vi "Target Deterministic Tasks.vi"(6 "rt fifo":refnum<k33>, 8 "Start Time (uSec)":u32) -> (0 "Stop":bool)   [LabVIEW 2018]
uses:
  Target Logging Cluster.ctl
  Target Sensors.ctl
  Target Telemetry Cluster.ctl
  COBRA-Libraries/Data Logging/COBRA Logging and Loop Timing Library.lvlib
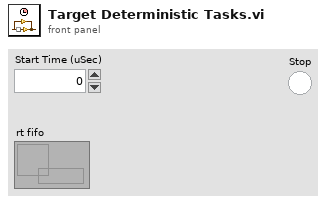
[diagram p1: front panel]
types:
  T1 = typedef "Target Logging Cluster.ctl" = cluster{"Valid for Logging?":bool, "Target Sensors":T2}
  T2 = typedef "Target Sensors.ctl" = cluster{"Raw Cable Force (N)":dbl, "Prosthesis Angle (deg)":dbl, "Main Clock Line (s)":dbl}
  T3 = enum16{"Manual Button Press", "External Voltage"}
  T4 = typedef "Target Telemetry Cluster.ctl" = cluster{"Target Sensors":T2}
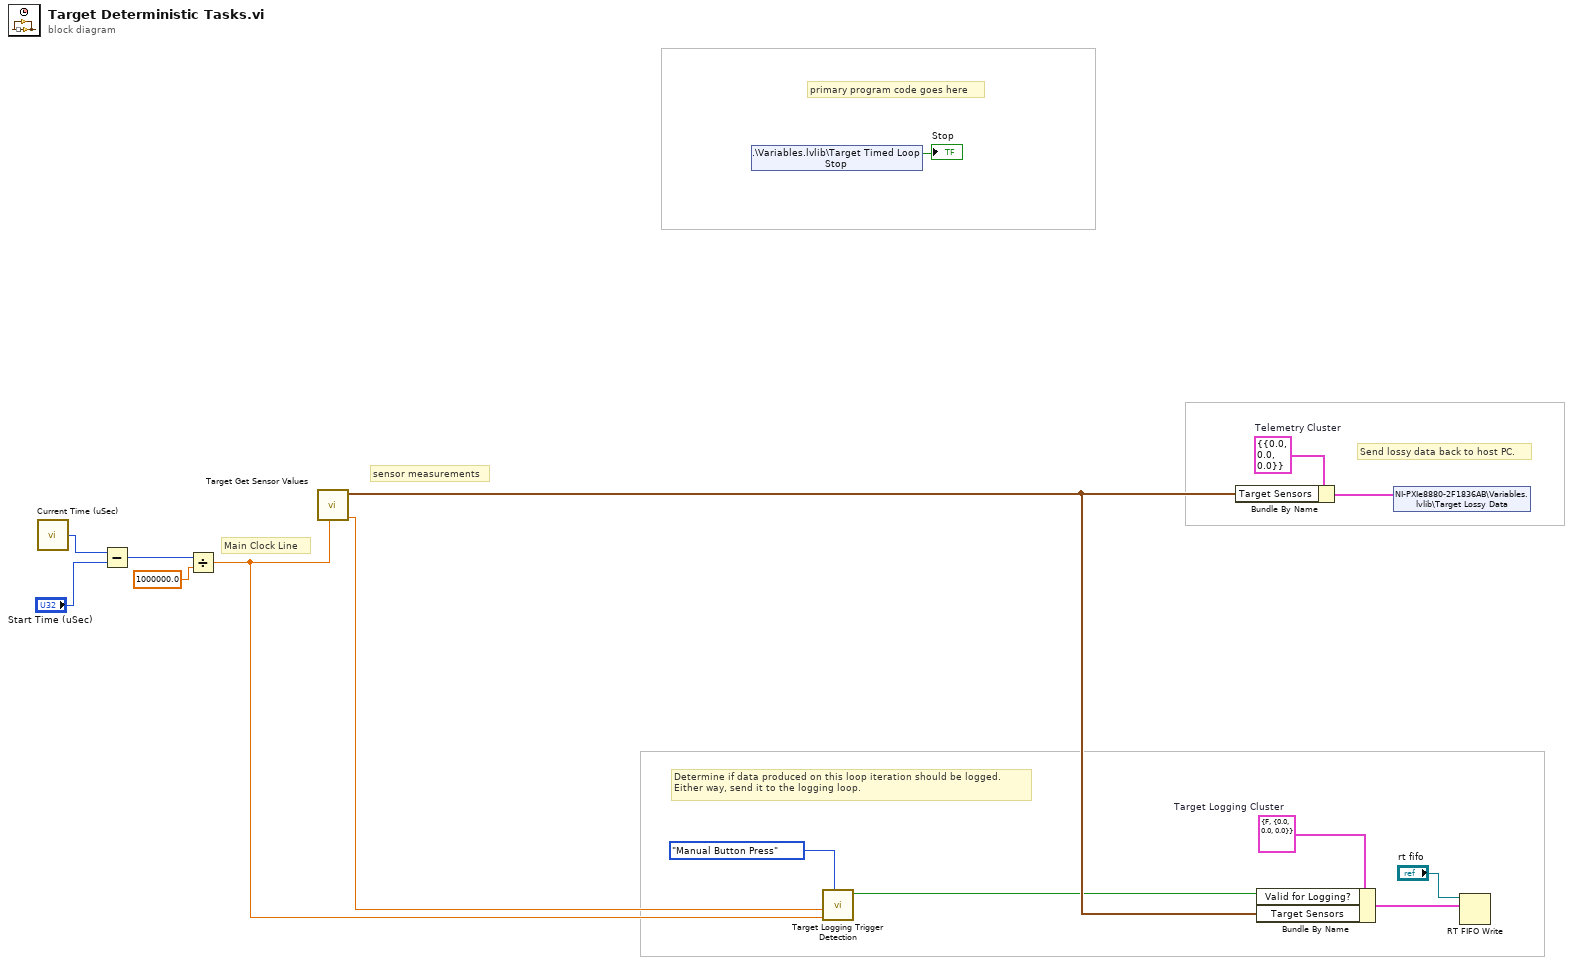
[diagram p0: block diagram]
diagram:
  w6 = T1 {"Valid for Logging?"=FALSE, "Target Sensors"={"Raw Cable Force (N)"=0.0, "Prosthesis Angle (deg)"=0.0, "Main Clock Line (s)"=0.0}}  # Target Logging Cluster
  w13 = T4 {"Target Sensors"={"Raw Cable Force (N)"=0.0, "Prosthesis Angle (deg)"=0.0, "Main Clock Line (s)"=0.0}}  # Telemetry Cluster
  # "primary program code goes here"
  # "sensor measurements"
  # "Main Clock Line"
  # "Send lossy data back to host PC."
  # "Determine if data produced on this loop iteration should be logged.\nEither way, send it to the logging loop."
  n1 = call "Current Time (uSec)"() -> ("Tick Count(uSec)"=w9:u32)
  n2 = Subtract(x=w9, y="Start Time (uSec)") -> (x-y=w11:u32)
  n3 = Divide(x=w11, y=1000000.0) -> (x/y=w4:dbl)
  n4 = call "Target Get Sensor Values.vi"("Main Clock Line (s)"=w4) -> ("Vicon Log Trigger"=w3:dbl, "Target Sensors"=w8:T2)  [unwired: 9 in]
  n5 = shared-variable ".\\Variables.lvlib\\Target Timed Loop Stop"() -> (→"Stop":bool)  [unwired: 1 in, 1 out]
  n6 = call "Target Logging Trigger Detection.vi"("Trigger Mode"=T3."Manual Button Press", "Main Clock Line (s)"=w4, "External Trigger Voltage"=w3) -> ("Valid for Logging?"=w1:bool)  [unwired: 8 in]
  n7 = Bundle By Name(cluster=w13, "Target Sensors"=w8) -> (w7:T4)
  n8 = Bundle By Name(cluster=w6, "Valid for Logging?"=w1, "Target Sensors"=w8) -> (w14:T1)
  n9 = shared-variable "NI-PXIe8880-2F1836AB\\Variables.lvlib\\Target Lossy Data"(w7) -> ()  [unwired: 1 in, 1 out]
  n10 = RT FIFO Write(0:"rt fifo", 1:w14) -> ()  [unwired: 3 in, 4 out]
